vi "Reset.vi"(8 "error in (no error)":errorcluster, 9 "Reset mode (5: Soft Reset)":u32(ring)=5 items=["No Reset", "Reset counter value (no mode change)", "Reset alarm", "Restart batch counter", "Reset counter value (counter off)", "Soft Reset"], 10 "Node (3)":u8=3 caption="Node" min=3 max=128 step=1, 11 "VISA resource name":refnum<visa-resource-name>) -> (0 "error out":errorcluster, 3 "VISA resource name out":refnum<visa-resource-name>)   [LabVIEW 2022 SP3, in "Bronkhorst FLOW-BUS.lvlib"]
doc: "Resets several values in the instrument. The VIs default action is performing a softreset on the device."
uses:
  Bronkhorst FLOW-BUS.lvlib
  Private/FLOW-BUS RW.ctl
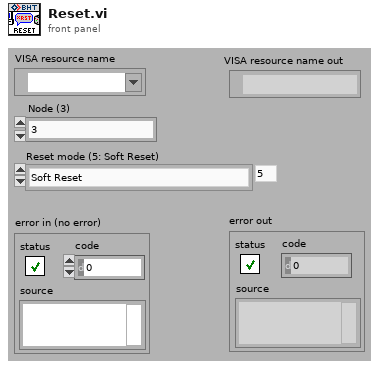
[diagram p1: front panel]
types:
  T1 = typedef "Bronkhorst FLOW-BUS.lvlib/FLOW-BUS RW.ctl" = cluster{"Node Address (3)":u8, "Communication Command":enum16{"Status message", "Send parameter with destination address and 00 response", "Send parameter with destination address", "Request parameter"}, "Process (0)":u16, "Parameter (0)":u16, "Data Type (0: Character)":enum16{"Character", "Integer", "Float or Long", "String"}, "Data for Char or Int (0)":u32, "Data for Float or Long (0)":sgl, "Data for String":string, "Length of Requested String (0)":u8}
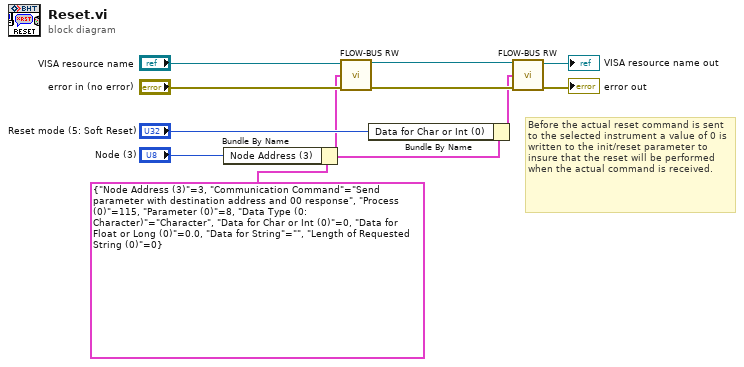
[diagram p0: block diagram]
diagram:
  # "Before the actual reset command is sent to the selected instrument a value of 0 is written to the init/reset parameter to insure that the reset will be performed when the actual command is received."
  n1 = Bundle By Name(cluster=T1 {"Node Address (3)"=3, "Communication Command"=enum."Send parameter with destination address and 00 response", "Process (0)"=115, "Parameter (0)"=8, "Data Type (0: Character)"=enum."Character", "Data for Char or Int (0)"=0, "Data for Float or Long (0)"=0.0, "Data for String"="", "Length of Requested String (0)"=0} ("FLOW-BUS Command Settings"), "Node Address (3)"="Node (3)") -> (w2:T1)
  n2 = call "FLOW-BUS RW.vi"("VISA resource name"="VISA resource name", "FLOW-BUS Command Settings"=w2, "error in (no error)"="error in (no error)") -> ("VISA resource name out"=w6:refnum<visa-resource-name>, "error out"=w7:errorcluster)  [unwired: 8 in, 3 out]
  n3 = Bundle By Name(cluster=w2, "Data for Char or Int (0)"="Reset mode (5: Soft Reset)") -> (w3:T1)
  n4 = call "FLOW-BUS RW.vi"("VISA resource name"=w6, "FLOW-BUS Command Settings"=w3, "error in (no error)"=w7) -> ("VISA resource name out"=→"VISA resource name out":refnum<visa-resource-name>, "error out"=→"error out":errorcluster)  [unwired: 8 in, 3 out]
